vi "SLSC_12201_AsynRTEngine.vi"(10 "Parameters":variant, 11 "Process":refnum<class "Process.lvclass">) -> ()   [LabVIEW 2015, in "SLSC-12201 DIO Engine.lvlib"]
uses:
  SLSC-12201 DIO Engine.lvlib
  <vilib>/NI/NIVS Inline Async API/_VS Inline Async API/Process/Process.lvclass
  Types/Async Engine State Control.ctl
  Shared/Compiled.Settings
  Shared/SLSC Dynamic Channel.ctl
  Shared/SLSC Dynamic Channel Type.ctl
  <vilib>/NI/NIVS Inline Async API/_VS Inline Async API/Process/Process.lvclass/Process.ctl
  <vilib>/NI/NIVS Inline Async API/_Data Access Engine/Access Type Classes/Read/Read.lvclass/Read.ctl
  <vilib>/NI/NIVS Inline Async API/_Data Access Engine/Access Type Classes/ReadWrite/ReadWrite.lvclass/ReadWrite.ctl
  <vilib>/NI/NIVS Inline Async API/_Data Access Engine/Access Type Classes/Write/Write.lvclass/Write.ctl
  <vilib>/NI/NIVS Inline Async API/_Data Access Engine/Data Access Engine/Methods/Read.Data.vi
  <vilib>/NI/NIVS Inline Async API/_Data Access Engine/Data Access Engine/Methods/Read.Data.Detect.vi
  <vilib>/NI/NIVS Inline Async API/_Data Access Engine/Data Access Engine/Methods/Write.Data.vi
  <vilib>/NI/NIVS Inline Async API/_Data Access Engine/Data Access Engine/Methods/ReadWrite.Data.vi
  <vilib>/NI/NIVS Inline Async API/_VS Inline Async API/Process/Data Member Access/Read Data Access.vi
  <vilib>/NI/NIVS Inline Async API/_VS Inline Async API/Error Handling Process/SubVIs/Error.ConvertArray.vi
  SLSC_Determine_Resource.vi
  <vilib>/NI/NIVS Inline Async API/_Data Access Engine/Access Type Classes/Read/Read.ProcessData.vi
  <vilib>/NI/NIVS Inline Async API/_Data Access Engine/Access Type Classes/Read/Read.ProcessData.Detect.vi
  <vilib>/NI/NIVS Inline Async API/_Data Access Engine/Access Type Classes/Write/Write.ProcessData.vi
  <vilib>/NI/NIVS Inline Async API/_Data Access Engine/Access Type Classes/ReadWrite/ReadWrite.ProcessData.vi
  <vilib>/SLSC/Close Session.vi
  <vilib>/SLSC/Execute Command.vi
  <vilib>/SLSC/Execute Phys Chan Command.vi
  <vilib>/SLSC/Execute Device Command.vi
  <vilib>/SLSC/Commit Properties.vi
  <vilib>/SLSC/Commit Properties for Devices.vi
  <vilib>/SLSC/Set Generic Property.vi
  <vilib>/SLSC/Set Generic Property (U64).vi
  <vilib>/SLSC/Set Generic Property (U32).vi
  <vilib>/SLSC/Set Generic Property (String).vi
  <vilib>/SLSC/Set Generic Property (I64).vi
  <vilib>/SLSC/Set Generic Property (I32).vi
  <vilib>/SLSC/Set Generic Property (DBL).vi
  <vilib>/SLSC/Set Generic Property (Bool).vi
  <vilib>/SLSC/Get Generic Property.vi
  <vilib>/SLSC/Get Generic Property (U64).vi
  <vilib>/SLSC/Get Generic Property (U32).vi
  <vilib>/SLSC/Get Generic Property (String).vi
  <vilib>/SLSC/Get Generic Property (I64).vi
  <vilib>/SLSC/Get Generic Property (I32).vi
  <vilib>/SLSC/Get Generic Property (DBL).vi
  <vilib>/SLSC/Get Generic Property (Bool).vi
  <vilib>/NI/NIVS Inline Async API/_Data Access Engine/Data Access Engine/Methods/Write.Lookup.vi
  <vilib>/NI/NIVS Inline Async API/_Data Access Engine/Data Access Engine/Methods/ReadWrite.Lookup.vi
  <vilib>/NI/NIVS Inline Async API/_Data Access Engine/Data Access Engine/Methods/Read.Lookup.vi
  Shared/Constants.vi
  <vilib>/NI/NIVS Inline Async API/_Data Access Engine/Data Access Engine/Data Access Engine.lvclass
  <vilib>/NI Veristand/Custom Device Tools/Custom Device Utility Library/Custom Device Utility Library.lvlib
  <vilib>/SLSC/SLSC.lvlib
  Shared/SLSC-12201 DIO Shared.lvlib
  System Explorer/SLSC-12201 DIO System Explorer.lvlib
panel:
  out "Async Engine Control":T1
  out "error IO":errorcluster
  in  "LoopRate(ms)":u32=50
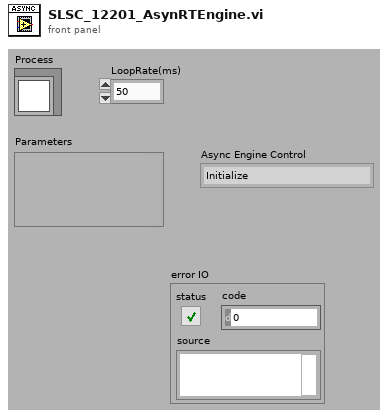
[diagram p1: front panel]
types:
  T1 = typedef "SLSC-12201 DIO Engine.lvlib/Async Engine State Control.ctl" = enum16{"Initialize", "Configure", "Run", "Reset", "Shutdown"}
  T2 = typedef "SLSC-12201 DIO Shared.lvlib/Compiled.Settings" = cluster{"Name":string, "SLSC IP Address":string, "Slot #":i32, "Configuration Data":cluster{"Properties":cluster{"Boolean Properties":cluster{"property":refnum<k21>, "Value":bool, "SLSC Item":refnum<k21>}[], "Double Properties":cluster{"property":refnum<k21>, "Double Write":dbl, "SLSC Item":refnum<k21>}[], "I32 Properties":cluster{"property":refnum<k21>, "Int32 Write":i32, "SLSC Item":refnum<k21>}[], "I64 Properties":cluster{"property":refnum<k21>, "Int64 Write":i64, "SLSC Item":refnum<k21>}[], "String Properties":cluster{"property":refnum<k21>, "String Write":string, "SLSC Item":refnum<k21>}[], "U32 Properties":cluster{"property":refnum<k21>, "UInt32 Write":u32, "SLSC Item":refnum<k21>}[], "U64 Properties":cluster{"property":refnum<k21>, "UInt64 Write":u64, "SLSC Item":refnum<k21>}[]}}, "SLSC Set Properties":T3[], "SLSC Get Properties":T3[], "SLSC Commands":T3[], "Username":string, "Password":string, "Support Modules":cluster{"Dev.ProductNumber":u32, "Dev.VendorNumber":u32}[]}
  T3 = typedef "SLSC-12201 DIO System Explorer.lvlib/SLSC Dynamic Channel.ctl" = cluster{"SLSC Item":string, "property":string, "Data Type":T4, "Value":variant}
  T4 = typedef "SLSC-12201 DIO System Explorer.lvlib/SLSC Dynamic Channel Type.ctl" = enum16{"Bool", "Double", "I32", "I64", "String", "U32", "U64", "EnumI32"}
  T5 = typedef "Data Access Engine.lvlib/Data Access Engine.lvclass/Read.DVR.ctl" = refnum<data-value>
  T6 = typedef "Data Access Engine.lvlib/Data Access Engine.lvclass/ReadWrite.DVR.ctl" = refnum<data-value>
  T7 = typedef "Data Access Engine.lvlib/Data Access Engine.lvclass/Write.DVR.ctl" = refnum<data-value>
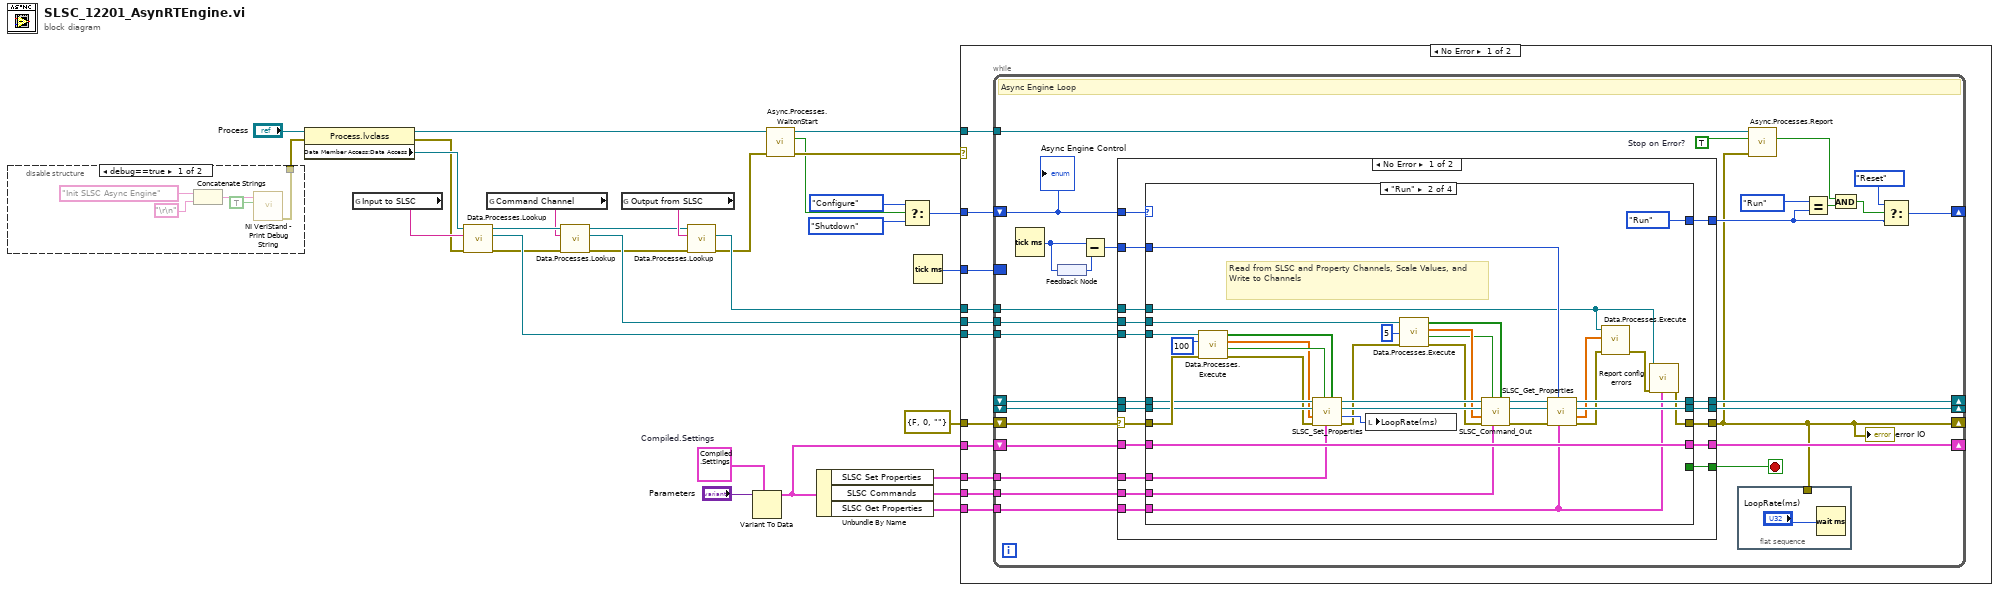
[diagram p0: block diagram]
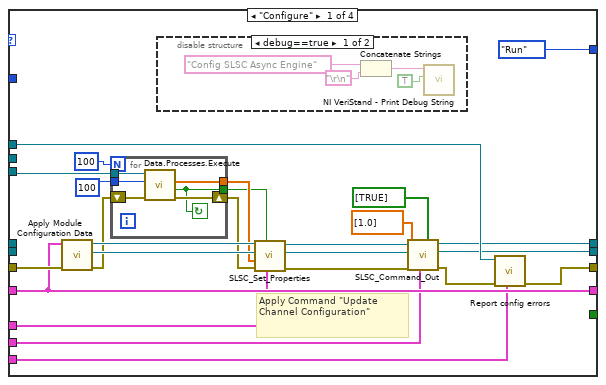
[diagram p3: hidden frame]
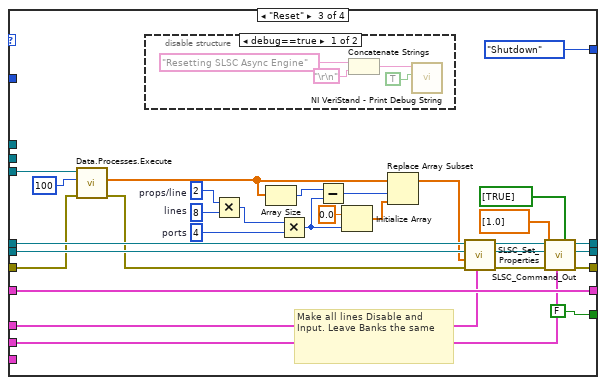
[diagram p5: hidden frame]
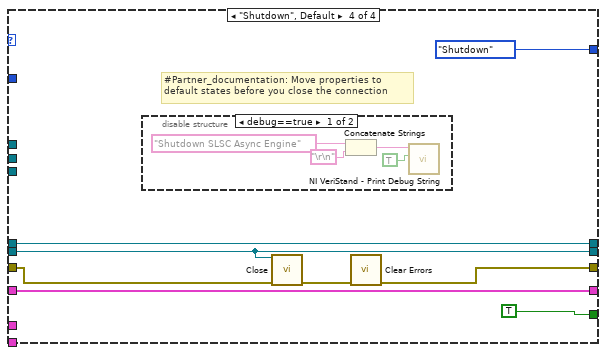
[diagram p7: hidden frame]
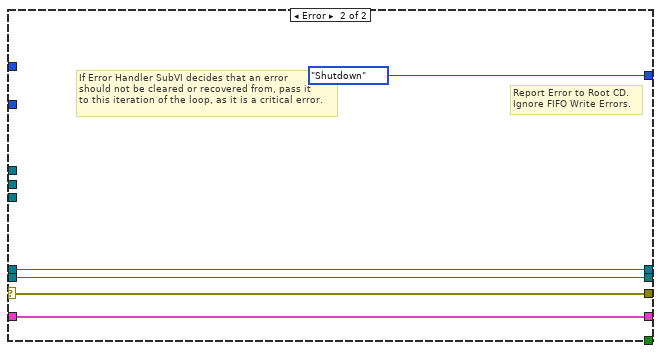
[diagram p9: hidden frame]
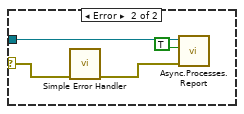
[diagram p10: hidden frame]
diagram:
  w23 = T2 {"Name"="", "SLSC IP Address"="", "Slot #"=0, "Configuration Data"={"Properties"={"Boolean Properties"=[], "Double Properties"=[], "I32 Properties"=[], "I64 Properties"=[], "String Properties"=[], "U32 Properties"=[], "U64 Properties"=[]}}, "SLSC Set Properties"=[], "SLSC Get Properties"=[], "SLSC Commands"=[], "Username"="", "Password"="", "Support Modules"=[]}  # Compiled.Settings
  n1 = disable-structure shown="debug==true" {
    disable-tunnel: [w31 _] -> w13
    frame condition #0 {
      n2 = Concatenate Strings("Init SLSC Async Engine" ("Message"), "\r\n") -> (w34:string)
      n3 = call <vilib>:"NI VeriStand - Print Debug String.vi"("Add to log file? (T)"=TRUE, "Message"=w34) -> ("error out"=w31:errorcluster)  [unwired: 9 in]
    }
    frame condition #1 (active) {
    }
  }
  n4 = property class="Process.lvclass"(reference="Process", error in=w13) -> (reference out=w25:refnum<class "Process.lvclass">, error out=w2:errorcluster, "Data Member Access:Data Access"=w3:refnum<class "Data Access Engine.lvclass">)
  n5 = global read "Constants.vi" "Input to SLSC"() -> (w15:string)
  n6 = call-poly <vilib>:"Data.Processes.Lookup.vi"("error in (no error)"=w2, "Name"=w15, "Data Access API in"=w3) -> ("error out"=w10:errorcluster, "Ref"=w28:T5, "Data Access API out"=w11:refnum<class "Data Access Engine.lvclass">)  [unwired: 5 in, 1 out]
  n7 = global read "Constants.vi" "Command Channel"() -> (w9:string)
  n8 = call-poly <vilib>:"Data.Processes.Lookup.vi"("error in (no error)"=w10, "Name"=w9, "Data Access API in"=w11) -> ("error out"=w5:errorcluster, "Ref"=w8:T6, "Data Access API out"=w4:refnum<class "Data Access Engine.lvclass">)  [unwired: 5 in, 1 out]
  n9 = global read "Constants.vi" "Output from SLSC"() -> (w16:string)
  n10 = call-poly <vilib>:"Data.Processes.Lookup.vi"("error in (no error)"=w5, "Name"=w16, "Data Access API in"=w4) -> ("error out"=w1:errorcluster, "Ref"=w27:T7)  [unwired: 5 in, 2 out]
  n11 = Variant To Data(type=w23, Variant="Parameters") -> (data=w18:T2)  [unwired: 1 in, 1 out]
  n12 = call <vilib>:"Async.Processes.WaitonStart.vi"("error in (no error)"=w1, "Process"=w25) -> ("error out"=w29:errorcluster, "Execute"=w22:bool, "Process out"=w30:refnum<class "Process.lvclass">)  [unwired: 7 in]
  n13 = Unbundle By Name(w18) -> ("SLSC Set Properties"=w17:T3[], "SLSC Commands"=w12:T3[], "SLSC Get Properties"=w6:T3[])
  n14 = Select(t=Async_Engine_State_Control."Configure", s=w22, f=Async_Engine_State_Control."Shutdown") -> (s? t:f=w19:T1)
  n15 = Tick Count (ms)() -> (millisecond timer value=w14:u32)
  n16 = case shown="No Error" w29 {
    selector: w29 -> [_ w217]
    tunnel: w30 -> [w46 w218]
    tunnel: w27 -> [w45 _]
    tunnel: w28 -> [w44 _]
    tunnel: w18 -> [w39 _]
    tunnel: errorcluster {"status"=FALSE, "code"=0, "source"=""} ("error constant") -> [w43 _]
    tunnel: w19 -> [w42 _]
    tunnel: w17 -> [w41 _]
    tunnel: w14 -> [w40 _]
    tunnel: w12 -> [w38 _]
    tunnel: w8 -> [w37 _]
    tunnel: w6 -> [w36 _]
    frame No Error {
      n17 = while {
        shift-right: [w47] -> _
        shift-left: w43 -> [w74]
        shift-right: [w48] -> _
        shift-left: w42 -> [w73]
        shift-right: [w72] -> _
        shift-left: w39 -> [w71]
        shift-right: [w70] -> _
        shift-left: _ -> [w69]
        tunnel: w44 -> [w68]
        tunnel: w45 -> [w67]
        tunnel: w46 -> [w66]
        tunnel: w41 -> [w65]
        shift-right: [w64] -> _
        shift-left: _ -> [w63]
        border: w40 -> [_]
        tunnel: w38 -> [w55]
        tunnel: w37 -> [w54]
        tunnel: w36 -> [w53]
        stop <- w58 stop-if-true
        w62 = TRUE  # Stop on Error?
        # "Async Engine Loop"
        n18 = Tick Count (ms)() -> (millisecond timer value=w61:u32)
        n19 = feedback-in #1(w61) -> ()
        n20 = feedback #1() -> (w60:u32)
        n21 = Subtract(x=w61, y=w60) -> (x-y=w59:u32)
        n22 = case shown="No Error" w74 {
          selector: w74 -> [w92 w211]
          tunnel: [w85 w211] -> w47
          tunnel: w73 -> [w93 _]
          tunnel: [w86 Async_Engine_State_Control."Shutdown"] -> w49
          tunnel: [w91 _] -> w58
          tunnel: [w90 w214] -> w72
          tunnel: w71 -> [w89 w214]
          tunnel: [w88 w213] -> w70
          tunnel: w69 -> [w87 w213]
          tunnel: w68 -> [w84 _]
          tunnel: w67 -> [w83 _]
          tunnel: w65 -> [w82 _]
          tunnel: [w81 w210] -> w64
          tunnel: w63 -> [w80 w210]
          tunnel: w59 -> [w79 _]
          tunnel: w55 -> [w78 _]
          tunnel: w54 -> [w77 _]
          tunnel: w53 -> [w76 _]
          frame No Error {
            n23 = case shown="\"Run\"" w93 {
              tunnel: w92 -> [w118 w160 w175 w198]
              tunnel: [w115 w130 w166 w201] -> w85
              tunnel: [Async_Engine_State_Control."Run" Async_Engine_State_Control."Run" Async_Engine_State_Control."Shutdown" Async_Engine_State_Control."Shutdown"] -> w86
              tunnel: [_ _ FALSE TRUE] -> w91
              tunnel: [w114 w163 w192 w204] -> w90
              tunnel: w89 -> [w114 w163 w192 w204]
              tunnel: [w112 w154 w167 w199] -> w88
              tunnel: w87 -> [_ w158 w186 w199]
              tunnel: w84 -> [w105 w161 w189 _]
              tunnel: w83 -> [w116 w131 _ _]
              tunnel: w82 -> [w101 w157 w188 _]
              tunnel: [w113 w155 w168 w200] -> w81
              tunnel: w80 -> [_ w156 w187 w200]
              tunnel: w79 -> [_ w151 _ _]
              tunnel: w78 -> [w95 w141 w165 _]
              tunnel: w77 -> [_ w149 _ _]
              tunnel: w76 -> [w108 w129 _ _]
              frame "Configure" {
                # "Apply Command \"Update Channel Configuration\""
                n24 = call "Apply Module Configuration Data.vi"("Error In"=w118, "Compiled.Settings"=w114) -> ("Error Out"=w100:errorcluster, "Device Session"=w106:refnum<k21>, "SLSC Module Name"=w107:refnum<k21>)  [unwired: 7 in]
                n25 = for {
                  N: 100 -> [_]
                  tunnel: w105 -> [w124]
                  tunnel: [w123] -> w104
                  tunnel: 100 ("timeout ms") -> [w122]
                  tunnel: [w119] -> w102
                  shift-right: [w120] -> w99
                  shift-left: w100 -> [w121]
                  stop <- w119 continue-if-true
                  n26 = call-poly <vilib>:"Data.Processes.Execute.vi"("error in (no error)"=w121, "timeout ms"=w122, "Ref"=w124) -> ("error out"=w120:errorcluster, "Timeout?"=w119:bool, "Values"=w123:dbl[])  [unwired: 6 in]
                }
                n27 = disable-structure shown="debug==true" {
                  frame condition #0 {
                    n28 = Concatenate Strings("Config SLSC Async Engine" ("Message"), "\r\n") -> (w126:string)
                    n29 = call <vilib>:"NI VeriStand - Print Debug String.vi"("Add to log file? (T)"=TRUE, "Message"=w126) -> ()  [unwired: 9 in, 1 out]
                  }
                  frame condition #1 (active) {
                  }
                }
                n30 = call "SLSC_Set_Properties.vi"("SLSC Dynamic Outputs"=w101, "Stop Updating?"=w102, "error in"=w99, "Values"=w104, "session in"=w106, "SLSC Module Name"=w107) -> ("error out"=w96:errorcluster, "session out"=w97:refnum<k21>, "SLSC Module Name"=w98:refnum<k21>)  [unwired: 2 in, 1 out]
                n31 = call "SLSC_Command_Out.vi"("Detect?"=bool[] [TRUE], "SLSC Dynamic Commands"=w95, "error in"=w96, "Values"=dbl[] [1.0], "session in"=w97, "SLSC Module Name"=w98) -> ("error out"=w109:errorcluster, "session out"=w112:refnum<k21>, "SLSC Module Name"=w113:refnum<k21>)  [unwired: 3 in]
                n32 = call "Report config errors.vi"("SLSC Dynamic Inputs"=w108, "error in (no error)"=w109, "Data Value Reference in"=w116) -> ("error out"=w115:errorcluster)  [unwired: 8 in]
              }
              frame "Run" {
                # "Read from SLSC and Property Channels, Scale Values, and Write to Channels"
                n33 = call-poly <vilib>:"Data.Processes.Execute.vi"("error in (no error)"=w160, "timeout ms"=100, "Ref"=w161) -> ("error out"=w140:errorcluster, "Timeout?"=w137:bool, "Values"=w134:dbl[], "Detect?"=w133:bool[])  [unwired: 5 in]
                n34 = call "SLSC_Set_Properties.vi"("Detect?"=w133, "SLSC Dynamic Outputs"=w157, "Stop Updating?"=w137, "error in"=w140, "Values"=w134, "session in"=w158, "SLSC Module Name"=w156) -> ("error out"=w139:errorcluster, "LoopRate(ms)"=w152:u32, "session out"=w146:refnum<k21>, "SLSC Module Name"=w147:refnum<k21>)  [unwired: 1 in]
                n35 = local write "LoopRate(ms)"(w152) -> ()
                n36 = call-poly <vilib>:"Data.Processes.Execute.vi"("error in (no error)"=w139, "timeout ms"=5, "Ref"=w149) -> ("error out"=w138:errorcluster, "Timeout?"=w136:bool, "Data"=w143:dbl[], "Detect?"=w135:bool[])  [unwired: 5 in]
                n37 = call "SLSC_Command_Out.vi"("Detect?"=w135, "SLSC Dynamic Commands"=w141, "Timeout?"=w136, "error in"=w138, "Values"=w143, "session in"=w146, "SLSC Module Name"=w147) -> ("error out"=w142:errorcluster, "session out"=w144:refnum<k21>, "SLSC Module Name"=w145:refnum<k21>)  [unwired: 2 in]
                n38 = call "SLSC_Get_Properties.vi"("SLSC Dynamic Inputs"=w129, "LoopDuration(ms)"=w151, "error in"=w142, "session in"=w144, "SLSC Module Name"=w145) -> ("error out"=w153:errorcluster, "Values"=w150:dbl[], "session out"=w154:refnum<k21>, "SLSC Module Name"=w155:refnum<k21>)  [unwired: 3 in]
                n39 = call-poly <vilib>:"Data.Processes.Execute.vi"("error in (no error)"=w153, "Values"=w150, "Ref"=w131) -> ("error out"=w132:errorcluster)  [unwired: 8 in]
                n40 = call "Report config errors.vi"("SLSC Dynamic Inputs"=w129, "error in (no error)"=w132, "Data Value Reference in"=w131) -> ("error out"=w130:errorcluster)  [unwired: 8 in]
              }
              frame "Reset" {
                w179 = 4  # ports
                w181 = 8  # lines
                w182 = 2  # props/line
                # "Make all lines Disable and Input. Leave Banks the same"
                n41 = call-poly <vilib>:"Data.Processes.Execute.vi"("error in (no error)"=w175, "timeout ms"=100, "Ref"=w189) -> ("error out"=w174:errorcluster, "Values"=w178:dbl[])  [unwired: 6 in, 1 out]
                n42 = disable-structure shown="debug==true" {
                  frame condition #0 {
                    n43 = Concatenate Strings("Resetting SLSC Async Engine" ("Message"), "\r\n") -> (w195:string)
                    n44 = call <vilib>:"NI VeriStand - Print Debug String.vi"("Add to log file? (T)"=TRUE, "Message"=w195) -> ()  [unwired: 9 in, 1 out]
                  }
                  frame condition #1 (active) {
                  }
                }
                n45 = Multiply(x=w182, y=w181) -> (x*y=w180:i32)
                n46 = Array Size(array=w178) -> (size(s)=w177:i32)
                n47 = Multiply(x=w180, y=w179) -> (x*y=w176:i32)
                n48 = Subtract(x=w177, y=w176) -> (x-y=w164:i32)
                n49 = Initialize Array(0.0 ("Default value"), w176) -> (w184:dbl[])
                n50 = Replace Array Subset(array=w178, new element=w184, index=w164) -> (w183:dbl[])
                n51 = call "SLSC_Set_Properties.vi"("SLSC Dynamic Outputs"=w188, "error in"=w174, "Values"=w183, "session in"=w186, "SLSC Module Name"=w187) -> ("error out"=w169:errorcluster, "session out"=w170:refnum<k21>, "SLSC Module Name"=w171:refnum<k21>)  [unwired: 3 in, 1 out]
                n52 = call "SLSC_Command_Out.vi"("Detect?"=bool[] [TRUE], "SLSC Dynamic Commands"=w165, "error in"=w169, "Values"=dbl[] [1.0], "session in"=w170, "SLSC Module Name"=w171) -> ("error out"=w166:errorcluster, "session out"=w167:refnum<k21>, "SLSC Module Name"=w168:refnum<k21>)  [unwired: 3 in]
              }
              frame "Shutdown", Default {
                # "#Partner_documentation: Move properties to \ndefault states before you close the connection"
                n53 = disable-structure shown="debug==true" {
                  frame condition #0 {
                    n54 = Concatenate Strings("Shutdown SLSC Async Engine" ("Message"), "\r\n") -> (w207:string)
                    n55 = call <vilib>:"NI VeriStand - Print Debug String.vi"("Add to log file? (T)"=TRUE, "Message"=w207) -> ()  [unwired: 9 in, 1 out]
                  }
                  frame condition #1 (active) {
                  }
                }
                n56 = call-poly <vilib>:"Close.vi"("session in"=w199, "error in (no error)"=w198) -> ("error out"=w202:errorcluster)  [unwired: 13 in]
                n57 = call <vilib>:"Clear Errors.vi"("error in (no error)"=w202) -> ("error out"=w201:errorcluster)  [unwired: 5 in, 1 out]
              }
            }
          }
          frame Error {
            # "If Error Handler SubVI decides that an error\nshould not be cleared or recovered from, pass it\nto this iteration of the loop, as it is a critical error."
            # "Report Error to Root CD.\nIgnore FIFO Write Errors."
          }
        }
        "error IO" <- w47
        n58 = flat-sequence {
          tunnel: w47 -> [_]
          frame #0 {
            n59 = Wait (ms)(milliseconds to wait="LoopRate(ms)") -> ()  [unwired: 1 out]
          }
        }
        n60 = call <vilib>:"Async.Processes.Report.vi"("Error"=w47, "Stop Async on Error?"=w62, "Process in"=w66) -> ("Stop"=w57:bool)  [unwired: 7 in, 1 out]
        n61 = Equal?(x=Async_Engine_State_Control."Run", y=w49) -> (x = y?=w51:bool)
        n62 = And(x=w57, y=w51) -> (x .and. y?=w52:bool)
        n63 = Select(t=Async_Engine_State_Control."Reset", s=w52, f=w49) -> (s? t:f=w48:T1)
        "Async Engine Control" <- w73
      }
    }
    frame Error {
      n64 = call <vilib>:"Simple Error Handler.vi"("error in (no error)"=w217) -> ("error out"=w215:errorcluster)  [unwired: 4 in, 4 out]
      n65 = call <vilib>:"Async.Processes.Report.vi"("Error"=w215, "Stop Async on Error?"=TRUE ("Stop on Error?"), "Process in"=w218) -> ()  [unwired: 7 in, 2 out]
    }
  }
